vi "绝缘电阻测试.vi"(11 "Channel":u16=81 format="%.0x") -> (3 "绝缘电阻":u16)   [LabVIEW 2020]
uses:
  D/Program Files (x86)/National Instruments/LabVIEW 2020/user.lib/PCANBasic/PCANBasic.lvlib
panel:
  out "function return 2":u32 format="%.0x"
  out "function return 3":u32 format="%.0x"
  out "function return":u32 format="%.0x"
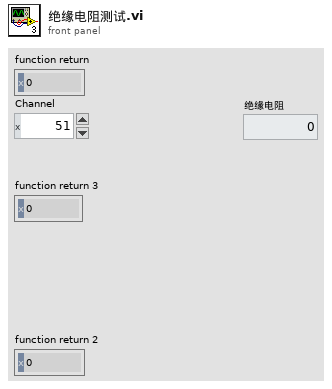
[diagram p1: front panel]
types:
  T1 = cluster{"ID":u32, "MSGTYPE":u8, "DLC":u8, "DATA[0]":u8, "DATA[1]":u8, "DATA[2]":u8, "DATA[3]":u8, "DATA[4]":u8, "DATA[5]":u8, "DATA[6]":u8, "DATA[7]":u8, "DATA[8]":u8, "DATA[9]":u8, "DATA[10]":u8, "DATA[11]":u8, "DATA[12]":u8, "DATA[13]":u8, "DATA[14]":u8, "DATA[15]":u8, "DATA[16]":u8, "DATA[17]":u8, "DATA[18]":u8, "DATA[19]":u8, "DATA[20]":u8, "DATA[21]":u8, "DATA[22]":u8, "DATA[23]":u8, "DATA[24]":u8, "DATA[25]":u8, "DATA[26]":u8, "DATA[27]":u8, "DATA[28]":u8, "DATA[29]":u8, "DATA[30]":u8, "DATA[31]":u8, "DATA[32]":u8, "DATA[33]":u8, "DATA[34]":u8, "DATA[35]":u8, "DATA[36]":u8, "DATA[37]":u8, "DATA[38]":u8, "DATA[39]":u8, "DATA[40]":u8, "DATA[41]":u8, "DATA[42]":u8, "DATA[43]":u8, "DATA[44]":u8, "DATA[45]":u8, "DATA[46]":u8, "DATA[47]":u8, "DATA[48]":u8, "DATA[49]":u8, "DATA[50]":u8, "DATA[51]":u8, "DATA[52]":u8, "DATA[53]":u8, "DATA[54]":u8, "DATA[55]":u8, "DATA[56]":u8, "DATA[57]":u8, "DATA[58]":u8, "DATA[59]":u8, "DATA[60]":u8, "DATA[61]":u8, "DATA[62]":u8, "DATA[63]":u8}
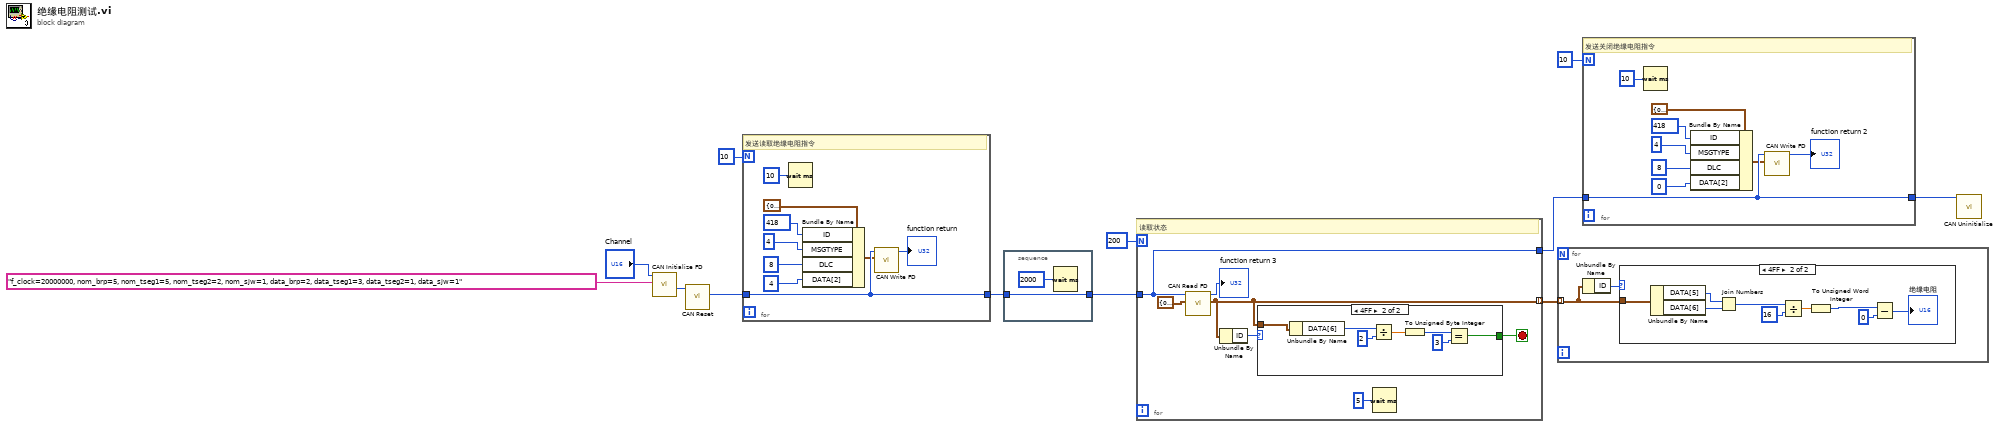
[diagram p0: block diagram]
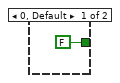
[diagram p3: hidden frame]
diagram:
  n1 = call "CAN Initialize FD.vi"("BitrateFD"="f_clock=20000000, nom_brp=5, nom_tseg1=5, nom_tseg2=2, nom_sjw=1, data_brp=2, data_tseg1=3, data_tseg2=1, data_sjw=1", "Channel"="Channel") -> ("Channel out"=w10:u16)  [unwired: 7 in, 2 out]
  n2 = call "CAN Reset.vi"("Channel in"=w10) -> ("Channel out"=w9:u16)  [unwired: 9 in, 1 out]
  n3 = for {
    N: 10 -> [_]
    tunnel: w9 -> [w19]
    tunnel: [w19] -> w7
    # "发送读取绝缘电阻指令"
    n4 = Wait (ms)(milliseconds to wait=u32 10 ("等待时间（毫秒）")) -> ()  [unwired: 1 out]
    n5 = Bundle By Name(cluster=T1 {"ID"=0, "MSGTYPE"=0, "DLC"=0, "DATA[0]"=0, "DATA[1]"=0, "DATA[2]"=0, "DATA[3]"=0, "DATA[4]"=0, "DATA[5]"=0, "DATA[6]"=0, "DATA[7]"=0, "DATA[8]"=0, "DATA[9]"=0, "DATA[10]"=0, "DATA[11]"=0, "DATA[12]"=0, "DATA[13]"=0, "DATA[14]"=0, "DATA[15]"=0, "DATA[16]"=0, "DATA[17]"=0, "DATA[18]"=0, "DATA[19]"=0, "DATA[20]"=0, "DATA[21]"=0, "DATA[22]"=0, "DATA[23]"=0, "DATA[24]"=0, "DATA[25]"=0, "DATA[26]"=0, "DATA[27]"=0, "DATA[28]"=0, "DATA[29]"=0, "DATA[30]"=0, "DATA[31]"=0, "DATA[32]"=0, "DATA[33]"=0, "DATA[34]"=0, "DATA[35]"=0, "DATA[36]"=0, "DATA[37]"=0, "DATA[38]"=0, "DATA[39]"=0, "DATA[40]"=0, "DATA[41]"=0, "DATA[42]"=0, "DATA[43]"=0, "DATA[44]"=0, "DATA[45]"=0, "DATA[46]"=0, "DATA[47]"=0, "DATA[48]"=0, "DATA[49]"=0, "DATA[50]"=0, "DATA[51]"=0, "DATA[52]"=0, "DATA[53]"=0, "DATA[54]"=0, "DATA[55]"=0, "DATA[56]"=0, "DATA[57]"=0, "DATA[58]"=0, "DATA[59]"=0, "DATA[60]"=0, "DATA[61]"=0, "DATA[62]"=0, "DATA[63]"=0} ("MessageBuffer"), "ID"=u32 418, "MSGTYPE"=u8 4, "DLC"=u8 8 ("ID"), "DATA[2]"=u8 4 ("ID")) -> (w13:T1)
    n6 = call "CAN Write FD.vi"("MessageBuffer"=w13, "Channel"=w19) -> ("function return"=→"function return":u32)  [unwired: 7 in, 2 out]
  }
  n7 = stacked-sequence {
    tunnel: w7 -> [w23]
    tunnel: [w23] -> w5
    frame #0 {
      n8 = Wait (ms)(milliseconds to wait=u32 2000 ("等待时间（毫秒）")) -> ()  [unwired: 1 out]
    }
  }
  n9 = for {
    N: 200 -> [_]
    tunnel: w5 -> [w29]
    tunnel: [w25] -> w4 mode=indexing
    tunnel: [w29] -> w2
    stop <- w24 stop-if-true
    # "读取状态"
    n10 = call "CAN Read FD.vi"("MessageBuffer"=T1 {"ID"=0, "MSGTYPE"=0, "DLC"=0, "DATA[0]"=0, "DATA[1]"=0, "DATA[2]"=0, "DATA[3]"=0, "DATA[4]"=0, "DATA[5]"=0, "DATA[6]"=0, "DATA[7]"=0, "DATA[8]"=0, "DATA[9]"=0, "DATA[10]"=0, "DATA[11]"=0, "DATA[12]"=0, "DATA[13]"=0, "DATA[14]"=0, "DATA[15]"=0, "DATA[16]"=0, "DATA[17]"=0, "DATA[18]"=0, "DATA[19]"=0, "DATA[20]"=0, "DATA[21]"=0, "DATA[22]"=0, "DATA[23]"=0, "DATA[24]"=0, "DATA[25]"=0, "DATA[26]"=0, "DATA[27]"=0, "DATA[28]"=0, "DATA[29]"=0, "DATA[30]"=0, "DATA[31]"=0, "DATA[32]"=0, "DATA[33]"=0, "DATA[34]"=0, "DATA[35]"=0, "DATA[36]"=0, "DATA[37]"=0, "DATA[38]"=0, "DATA[39]"=0, "DATA[40]"=0, "DATA[41]"=0, "DATA[42]"=0, "DATA[43]"=0, "DATA[44]"=0, "DATA[45]"=0, "DATA[46]"=0, "DATA[47]"=0, "DATA[48]"=0, "DATA[49]"=0, "DATA[50]"=0, "DATA[51]"=0, "DATA[52]"=0, "DATA[53]"=0, "DATA[54]"=0, "DATA[55]"=0, "DATA[56]"=0, "DATA[57]"=0, "DATA[58]"=0, "DATA[59]"=0, "DATA[60]"=0, "DATA[61]"=0, "DATA[62]"=0, "DATA[63]"=0}, "Channel"=w29) -> ("MessageBuffer out"=w25:T1, "function return"=→"function return 3":u32)  [unwired: 6 in, 2 out]
    n11 = Unbundle By Name(w25) -> ("ID"=w26:u32)
    n12 = case shown="4FF" w26 {
      tunnel: w25 -> [_ w38]
      tunnel: [FALSE w34] -> w24
      frame 0, Default {
      }
      frame 1279 {
        n13 = Unbundle By Name(w38) -> ("DATA[6]"=w37:u8)
        n14 = Divide(x=w37, y=u8 2) -> (x/y=w32:dbl)
        n15 = To Unsigned Byte Integer(number=w32) -> (unsigned 8bit integer=w33:u8)
        n16 = Equal?(x=w33, y=u8 3) -> (x = y?=w34:bool)
      }
    }
    n17 = Wait (ms)(milliseconds to wait=u32 5 ("等待时间（毫秒）")) -> ()  [unwired: 1 out]
  }
  n18 = for {
    tunnel: w4 -> [w39] mode=indexing
    n19 = Unbundle By Name(w39) -> ("ID"=w40:u32)
    n20 = case shown="4FF" w40 {
      tunnel: w39 -> [_ w49]
      frame 0, Default {
      }
      frame 1279 {
        n21 = Unbundle By Name(w49) -> ("DATA[5]"=w47:u8, "DATA[6]"=w46:u8)
        n22 = Join Numbers(hi=w47, lo=w46) -> ((hi.lo)=w45:u16)
        n23 = Divide(x=w45, y=u8 16) -> (x/y=w43:dbl)
        n24 = To Unsigned Word Integer(number=w43) -> (unsigned 16bit integer=w42:u16)
        n25 = Subtract(x=w42, y=u16 0) -> (x-y=→"绝缘电阻":u16)
      }
    }
  }
  n26 = for {
    N: 10 -> [_]
    tunnel: w2 -> [w56]
    tunnel: [w56] -> w1
    # "发送关闭绝缘电阻指令"
    n27 = Wait (ms)(milliseconds to wait=u32 10 ("等待时间（毫秒）")) -> ()  [unwired: 1 out]
    n28 = Bundle By Name(cluster=T1 {"ID"=0, "MSGTYPE"=0, "DLC"=0, "DATA[0]"=0, "DATA[1]"=0, "DATA[2]"=0, "DATA[3]"=0, "DATA[4]"=0, "DATA[5]"=0, "DATA[6]"=0, "DATA[7]"=0, "DATA[8]"=0, "DATA[9]"=0, "DATA[10]"=0, "DATA[11]"=0, "DATA[12]"=0, "DATA[13]"=0, "DATA[14]"=0, "DATA[15]"=0, "DATA[16]"=0, "DATA[17]"=0, "DATA[18]"=0, "DATA[19]"=0, "DATA[20]"=0, "DATA[21]"=0, "DATA[22]"=0, "DATA[23]"=0, "DATA[24]"=0, "DATA[25]"=0, "DATA[26]"=0, "DATA[27]"=0, "DATA[28]"=0, "DATA[29]"=0, "DATA[30]"=0, "DATA[31]"=0, "DATA[32]"=0, "DATA[33]"=0, "DATA[34]"=0, "DATA[35]"=0, "DATA[36]"=0, "DATA[37]"=0, "DATA[38]"=0, "DATA[39]"=0, "DATA[40]"=0, "DATA[41]"=0, "DATA[42]"=0, "DATA[43]"=0, "DATA[44]"=0, "DATA[45]"=0, "DATA[46]"=0, "DATA[47]"=0, "DATA[48]"=0, "DATA[49]"=0, "DATA[50]"=0, "DATA[51]"=0, "DATA[52]"=0, "DATA[53]"=0, "DATA[54]"=0, "DATA[55]"=0, "DATA[56]"=0, "DATA[57]"=0, "DATA[58]"=0, "DATA[59]"=0, "DATA[60]"=0, "DATA[61]"=0, "DATA[62]"=0, "DATA[63]"=0} ("MessageBuffer"), "ID"=u32 418, "MSGTYPE"=u8 4, "DLC"=u8 8 ("ID"), "DATA[2]"=u8 0 ("ID")) -> (w50:T1)
    n29 = call "CAN Write FD.vi"("MessageBuffer"=w50, "Channel"=w56) -> ("function return"=→"function return 2":u32)  [unwired: 7 in, 2 out]
  }
  n30 = call "CAN Uninitialize.vi"("Channel"=w1) -> ()  [unwired: 10 in, 1 out]
